vi "demod.vi"(5 "Sync Word Length":i32, 7 "Preamble Length":i32, 8 "error in (no error)":errorcluster, 10 "input complex waveform":cluster{"t0":dbl, "dt":dbl, "Y":cdb[]}, 11 "Modulation Parameters In":T1={"RX Parameters"={"RX Oversample Factor"=4.0, "RX Sample Rate"=4000000.0, "Synchronization Options"={"Synchronization Method"=enum."Fixed Offset", "Symbol Timing Recovery Method "=enum."MT Allign To Ideal Symbols", "Fixed Offset"=0.0, "Frame Detection Method"=enum."", "Correct Frequency Offset"=FALSE}, "Channel Estimation/Equalization Parameters"={"Equalization Method"=enum."", "Channel Estimate Length"=0.0, "Equalizer Length"=0.0, "Equalizer Delay"=0.0}}, "TX/RX Shared Parameters"={"Modulation Type"=enum."OOK", "Packet Length"=128, "# of Iterations"=0.0, "Pulse Shaping Parameters"={"Pulse Shaping Filter"=enum."none", "Filter Length (symbols)"=32, "Filter Parameter"=0.8, "modulation type"=enum."FSK"}, "Header/Tail Control Information"={"Training Sequence Type"=enum."", "Zero Pad Length"=0.0}}}) -> (0 "error out":errorcluster, 2 "Received Bit Sequence":i32[](array[numeric]), 3 "Modulation Parameters Out":T1={"RX Parameters"={"RX Oversample Factor"=4.0, "RX Sample Rate"=4000000.0, "Synchronization Options"={"Synchronization Method"=enum."Fixed Offset", "Symbol Timing Recovery Method "=enum."MT Allign To Ideal Symbols", "Fixed Offset"=0.0, "Frame Detection Method"=enum."", "Correct Frequency Offset"=FALSE}, "Channel Estimation/Equalization Parameters"={"Equalization Method"=enum."", "Channel Estimate Length"=0.0, "Equalizer Length"=0.0, "Equalizer Delay"=0.0}}, "TX/RX Shared Parameters"={"Modulation Type"=enum."OOK", "Packet Length"=128, "# of Iterations"=0.0, "Pulse Shaping Parameters"={"Pulse Shaping Filter"=enum."none", "Filter Length (symbols)"=32, "Filter Parameter"=0.8, "modulation type"=enum."FSK"}, "Header/Tail Control Information"={"Training Sequence Type"=enum."", "Zero Pad Length"=0.0}}})   [LabVIEW 2012]
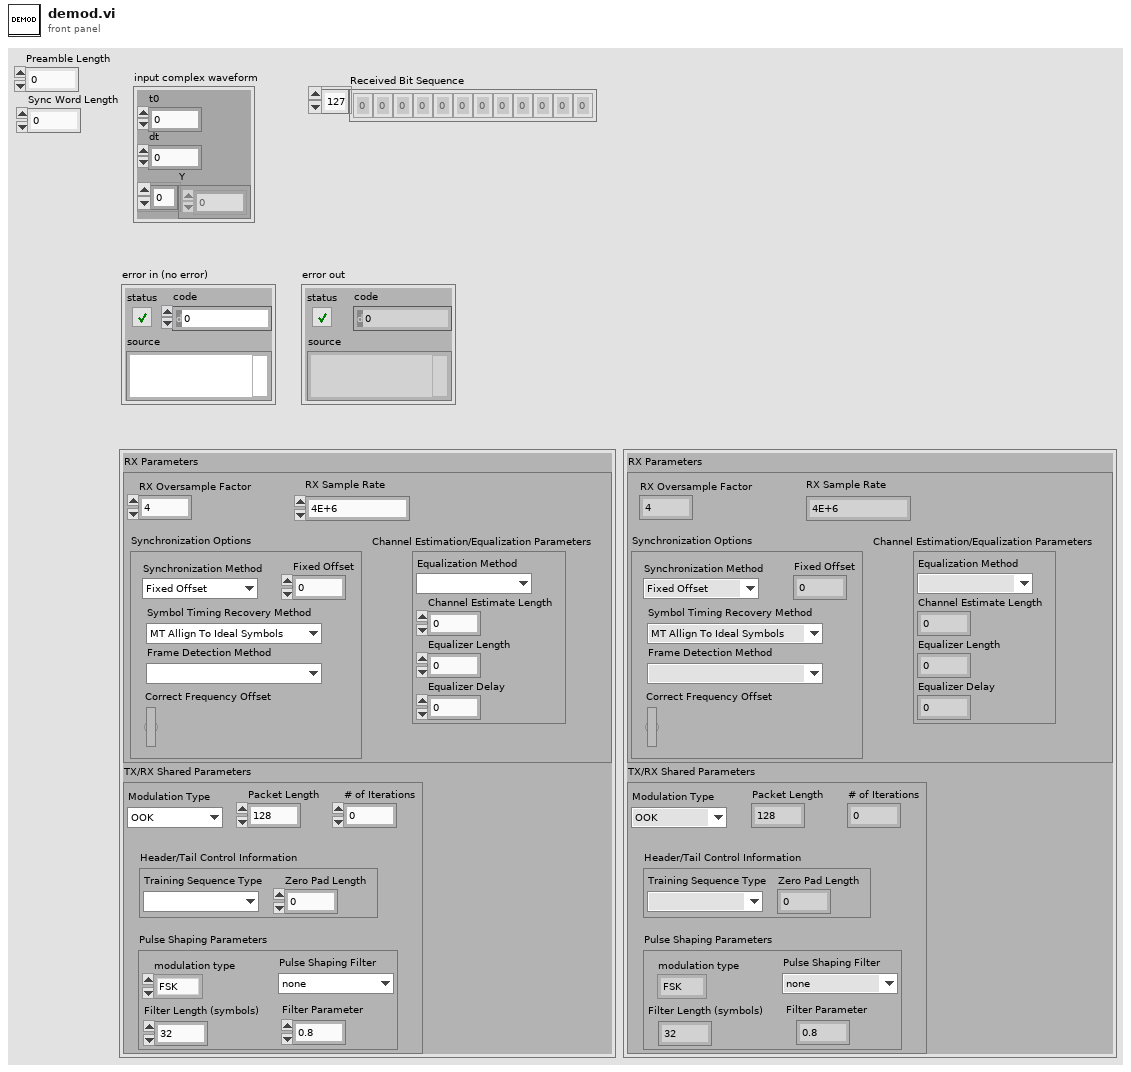
[diagram p1: front panel]
types:
  T1 = cluster{"RX Parameters":cluster{"RX Oversample Factor":dbl, "RX Sample Rate":dbl, "Synchronization Options":cluster{"Synchronization Method":enum16{"Fixed Offset", "Timing Estimation", "Joint Timing and Channel Estimation"}, "Symbol Timing Recovery Method ":enum16{"MT Allign To Ideal Symbols", "Maximum Energy", "Early-Late Gate", "Gardner", "Fixed Offset"}, "Fixed Offset":dbl, "Frame Detection Method":enum16{""}, "Correct Frequency Offset":bool}, "Channel Estimation/Equalization Parameters":cluster{"Equalization Method":enum16{""}, "Channel Estimate Length":dbl, "Equalizer Length":dbl, "Equalizer Delay":dbl}}, "TX/RX Shared Parameters":cluster{"Modulation Type":enum16{"OOK", "FSK"}, "Packet Length":i32, "# of Iterations":dbl, "Pulse Shaping Parameters":cluster{"Pulse Shaping Filter":enum16{"none", "Raised Cosine", "Root Raised Cos", "Gaussian"}, "Filter Length (symbols)":i32, "Filter Parameter":dbl, "modulation type":enum16{"FSK", "PSK", "QAM", "MSK", "PAM", "ASK", "CPM"}}, "Header/Tail Control Information":cluster{"Training Sequence Type":enum16{""}, "Zero Pad Length":dbl}}}
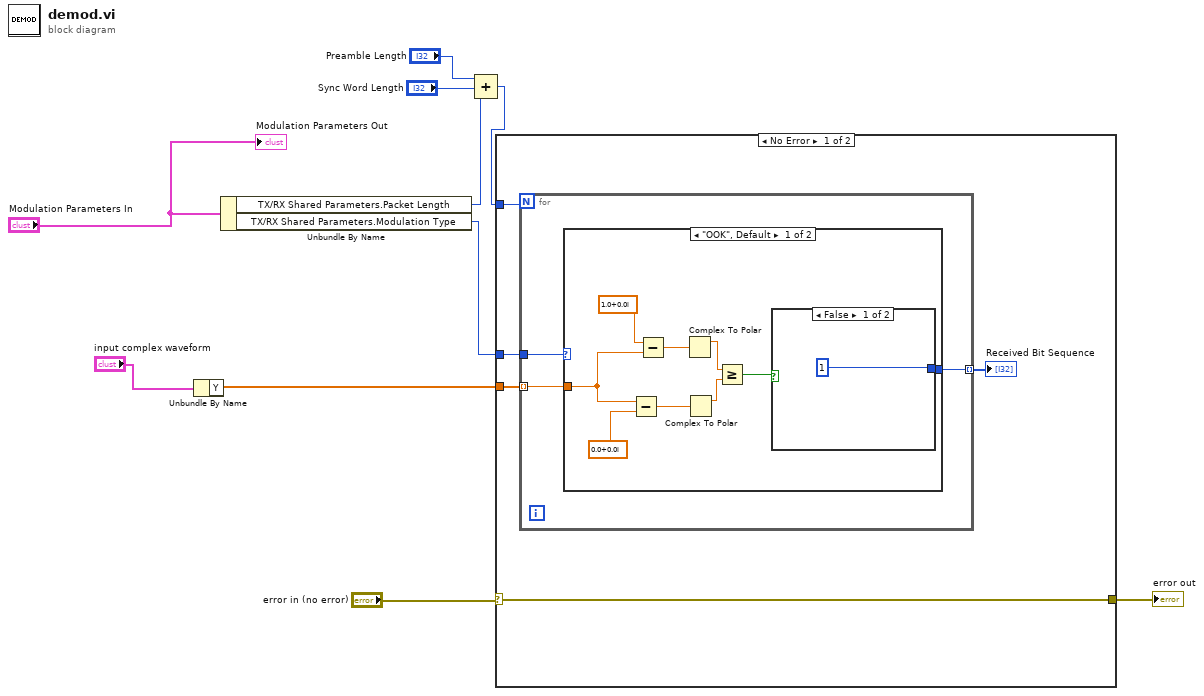
[diagram p0: block diagram]
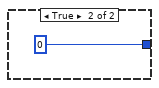
[diagram p2: hidden frame]
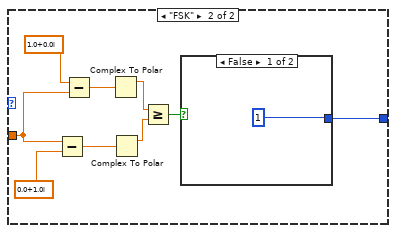
[diagram p3: hidden frame]
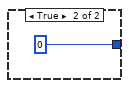
[diagram p4: hidden frame]
diagram:
  n1 = Unbundle By Name("input complex waveform") -> ("Y"=w6:cdb[])
  n2 = Unbundle By Name("Modulation Parameters In") -> ("TX/RX Shared Parameters.Packet Length"=w4:i32, "TX/RX Shared Parameters.Modulation Type"=w10:enum16{"OOK", "FSK"})
  n3 = Compound Arithmetic op=ADD("Preamble Length", "Sync Word Length", w4) -> (w3:i32)
  n4 = case shown="No Error" "error in (no error)" {
    selector: "error in (no error)" -> [w11 w41]
    tunnel: w3 -> [w15 _]
    tunnel: w10 -> [w14 _]
    tunnel: w6 -> [w13 _]
    tunnel: [w11 w41] -> w8
    frame No Error {
      n5 = for {
        N: w15 -> [_]
        tunnel: w14 -> [w18]
        tunnel: w13 -> [w17] mode=indexing
        tunnel: [w16] -> w12 mode=indexing
        n6 = case shown="\"OOK\", Default" w18 {
          tunnel: w17 -> [w21 w37]
          tunnel: [w19 w30] -> w16
          frame "OOK", Default {
            n7 = Subtract(x=w21, y=cdb 0.0+0.0i) -> (x-y=w24:cdb)
            n8 = Subtract(x=cdb 1.0+0.0i, y=w21) -> (x-y=w25:cdb)
            n9 = Complex To Polar(r * e^(i*theta)=w25) -> (r=w23:dbl)  [unwired: 1 out]
            n10 = Complex To Polar(r * e^(i*theta)=w24) -> (r=w22:dbl)  [unwired: 1 out]
            n11 = Greater Or Equal?(x=w23, y=w22) -> (x >= y?=w20:bool)
            n12 = case shown="False" w20 {
              tunnel: [1 0] -> w19
              frame False {
              }
              frame True {
              }
            }
          }
          frame "FSK" {
            n13 = Subtract(x=w37, y=cdb 0.0+1.0i) -> (x-y=w34:cdb)
            n14 = Subtract(x=cdb 1.0+0.0i, y=w37) -> (x-y=w35:cdb)
            n15 = Complex To Polar(r * e^(i*theta)=w35) -> (r=w32:dbl)  [unwired: 1 out]
            n16 = Complex To Polar(r * e^(i*theta)=w34) -> (r=w31:dbl)  [unwired: 1 out]
            n17 = Greater Or Equal?(x=w32, y=w31) -> (x >= y?=w33:bool)
            n18 = case shown="False" w33 {
              tunnel: [1 0] -> w30
              frame False {
              }
              frame True {
              }
            }
          }
        }
      }
      "Received Bit Sequence" <- w12
    }
    frame Error {
    }
  }
  "error out" <- w8
  "Modulation Parameters Out" <- "Modulation Parameters In"
